vi "Destroy XML Editor.vi"(8 "error in (no error)":errorcluster, 11 "Project XML Editor in":refnum<class "Project XML Editor.lvclass">) -> (0 "error out":errorcluster)   [LabVIEW 2019, in "LVLIBP CD XML Updater.lvlib" / "Project XML Editor.lvclass"]
uses:
  Project XML Editor.lvclass
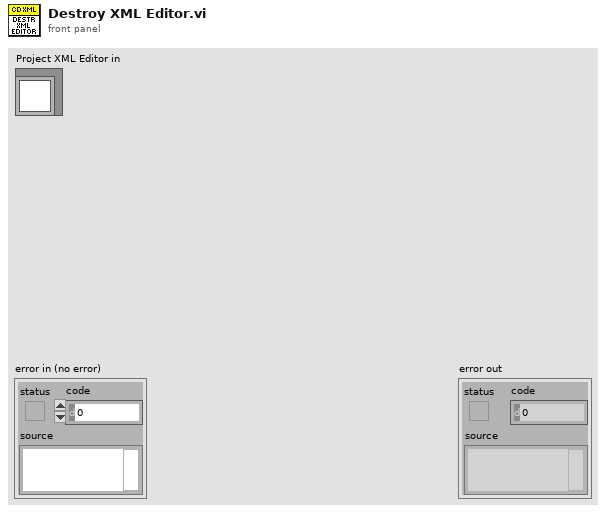
[diagram p1: front panel]
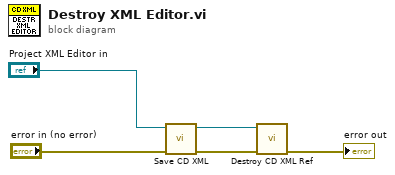
[diagram p0: block diagram]
diagram:
  n1 = call "Save CD XML.vi"("error in (no error)"="error in (no error)", "Project XML Editor in"="Project XML Editor in") -> ("error out"=w2:errorcluster, "Project XML Editor out"=w3:refnum<class "Project XML Editor.lvclass">)  [unwired: 8 in]
  n2 = call "Destroy CD XML Ref.vi"("error in (no error)"=w2, "Project XML Editor in"=w3) -> ("error out"=→"error out":errorcluster)  [unwired: 9 in]
